vi "Clean.vi"   [LabVIEW 2018, in "Scripts.lvlib"]
uses:
  Scripts.lvlib
  <vilib>/Field R&D Services/Labricator/Toolkit/Labricator.lvlib
panel:
  # "Overview: Deletes the artifacts for building and packaging\nRequirements: LabVIEW\nInstructions: Run this VI.\n\nDeletes the \"builds\" and \"target\" folders if they exist in the project root. Use with caution."
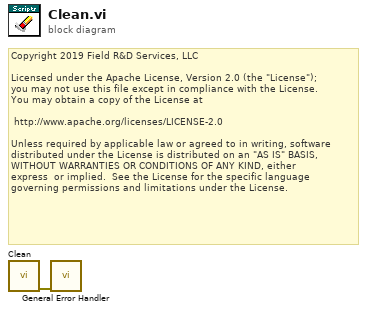
[diagram p0: block diagram]
diagram:
  # "Copyright 2019 Field R&D Services, LLC\n\nLicensed under the Apache License, Version 2.0 (the \"License\");\nyou may not use this file except in compliance with the License.\nYou may obtain a copy of the License at\n\n\thttp://www.apache.org/licenses/LICENSE-2.0\n\nUnless required by applicable law or agreed to in writing, software\ndistributed under the License is distributed on an \"AS IS\" BASIS,\nWITHOUT WARRANTIES OR CONDITIONS OF ANY KIND, either \nexpress  or implied.  See the License for the specific language \ngoverning permissions and limitations under the License."
  n1 = call <vilib>:"Clean.vi"() -> ("Error Out"=w1:errorcluster)  [unwired: 11 in]
  n2 = call <vilib>:"General Error Handler.vi"("error in (no error)"=w1) -> ()  [unwired: 10 in, 5 out]
